vi "Open.vi"(8 "error in (no error)":errorcluster, 9 "I2C Slave Address (4)":u8=4, 10 "I2C Channel (1)":u8=1, 11 "LINX Resource":T1={"IO"=enum."Local", "Interface"=enum."Serial", "LINX Device Config"={"Interface"=enum."Serial", "COM Port"="COM13", "TCP Configuration"={"IP Address"="", "Port"=0}, "Device Family"=1, "Device ID"=1, "Device Name"="myRIO-1900", "TCP Ref"=refnum, "Channels"={"DI"=[0, 1, 2, 3, 4, 5, 6, 7, 8, 9, 10, 11, 12, 13, 14, 15, 16, 17, 18, 19, 20, 21, 22, 23, 24, 25, 26, 27, 28, 29, 30, 31, 32, 33, 34, 35, 36, 37, 38, 39, 40, 41, 42, 43, 44, 45, 46], "DO"=[0, 1, 2, 3, 4, 5, 6, 7, 8, 9, 10, 11, 12, 13, 14, 15, 16, 17, 18, 19, 20, 21, 22, 23, 24, 25, 26, 27, 28, 29, 30, 31, 32, 33, 34, 35, 36, 37, 38, 39, 40, 41, 42, 43, 44, 45, 46], "AI"=[0, 1, 2, 3, 4, 5, 6, 7, 8, 9, 10, 11], "AO"=[], "PWM"=[3, 5, 6, 9, 10], "QE"=[], "UART"=[0, 1], "I2C 2"=[0], "SPI"=[0], "CAN"=[], "Servo"=[], "AI Ref (V)"=0.0, "AI Resolution (Bits)"=0, "AO Ref (V)"=0.0, "AO Resolution (Bits)"=0}}}) -> (0 "error out":errorcluster, 3 "LINX GrovePi out":refnum<class "LinxGrovePi.lvclass">)   [LabVIEW 2014, in "LinxGrovePi.lvclass"]
doc: "Configures the LINX Resource to use for I2C and opens the I2C channel and sets the slave address of the GrovePi.\n\nUse the LINX Resource after LINX has been opened."
uses:
  LinxGrovePi/LinxGrovePi.lvclass
  <vilib>/MakerHub/LINX/Private/Type Defs/LINX Ref.ctl
  <vilib>/MakerHub/LINX/Private/Type Defs/Platform.ctl
  <vilib>/MakerHub/LINX/Private/Type Defs/Interface.ctl
  <vilib>/MakerHub/LINX/Private/Device/Type Defs/LINX Device Config.ctl
  <vilib>/MakerHub/LINX/Private/Device/Type Defs/TCP Config.ctl
  <vilib>/MakerHub/LINX/Private/Device/Type Defs/Channels.ctl
  LinxGrovePi/LinxGrovePi.lvclass/LinxGrovePi.ctl
  I2C/I2C_Linx/LinxI2C.lvclass
  <vilib>/MakerHub/LINX/LMH-LINX.lvlib
  <vilib>/MakerHub/LINX/Private/Device/Device.lvlib
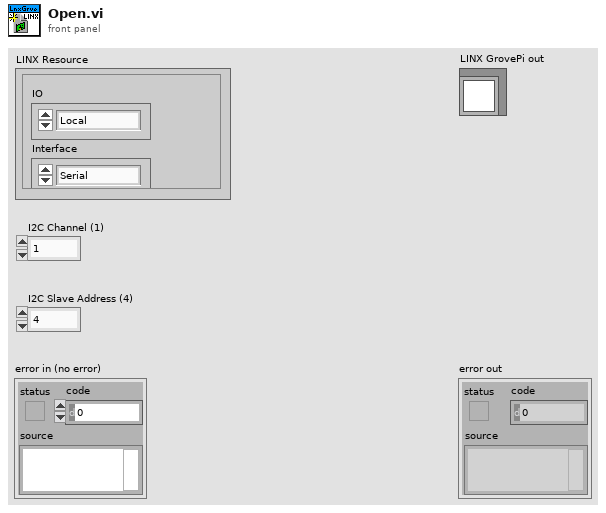
[diagram p1: front panel]
types:
  T1 = typedef "LMH-LINX.lvlib/LINX Ref.ctl" = cluster{"IO":T2, "Interface":T3, "LINX Device Config":T4}
  T2 = typedef "LMH-LINX.lvlib/Platform.ctl" = enum16{"Remote", "Local"}
  T3 = typedef "LMH-LINX.lvlib/Interface.ctl" = enum16{"Serial", "TCP"}
  T4 = typedef "LMH-LINX.lvlib/Device.lvlib/LINX Device Config.ctl" = cluster{"Interface":T3, "COM Port":refnum<visa-resource-name>, "TCP Configuration":T5, "Device Family":u8, "Device ID":u8, "Device Name":string, "TCP Ref":refnum<k5>, "Channels":T6}
  T5 = typedef "LMH-LINX.lvlib/Device.lvlib/TCP Config.ctl" = cluster{"IP Address":string, "Port":u16}
  T6 = typedef "LMH-LINX.lvlib/Channels.ctl" = cluster{"DI":u8[], "DO":u8[], "AI":u8[], "AO":u8[], "PWM":u8[], "QE":u8[], "UART":u8[], "I2C 2":u8[], "SPI":u8[], "CAN":u8[], "Servo":u8[], "AI Ref (V)":dbl, "AI Resolution (Bits)":u8, "AO Ref (V)":dbl, "AO Resolution (Bits)":u8}
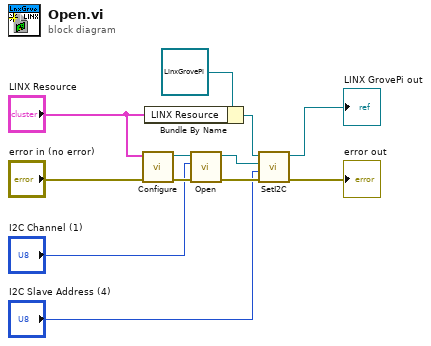
[diagram p0: block diagram]
diagram:
  n1 = call "Configure.vi"("error in (no error)"="error in (no error)", "LINX Resource"="LINX Resource") -> ("error out"=w11:errorcluster, "I2C Linx out"=w10:refnum<class "LinxI2C.lvclass">)  [unwired: 8 in]
  n2 = Bundle By Name(cluster=refnum<class "LinxGrovePi.lvclass"> refnum ("Linx GrovePi"), "LINX Resource"="LINX Resource") -> (w3:refnum<class "LinxGrovePi.lvclass">)
  n3 = call-dynamic "Open.vi"("error in (no error)"=w11, "I2C Channel"="I2C Channel (1)", "I2C Linx in"=w10) -> ("error out"=w9:errorcluster, "I2C Linx out"=w8:refnum<class "LinxI2C.lvclass">)  [unwired: 7 in]
  n4 = call-dynamic "SetI2C.vi"("error in (no error)"=w9, "I2C Slave Address"="I2C Slave Address (4)", "I2C"=w8, "GrovePi in"=w3) -> ("error out"=→"error out":errorcluster, "GrovePi out"=→"LINX GrovePi out":refnum<class "LinxGrovePi.lvclass">)  [unwired: 6 in]
